vi "UEvent_MEASURE_SEQ1_CLEAN_UP_DAQ.vi"(6 "USB  in":tag, 9 "Vout  - Vbat profile":enum16{"3.8VDC", "2.9VDC", "By Pass", "4.0VDC"}(ring), 10 "Range - Shunts in":T1, 11 "TASK IN":refnum<k21>) -> (0 "error out":errorcluster, 1 "DevSerialNum":u32, 7 "Power ON/OFF":bool)   [LabVIEW 2015]
uses:
  Range_Shunt_selector.ctl
  <resource>/objmgr/daqmx.rc
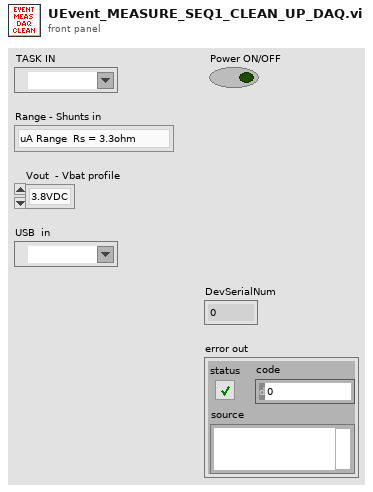
[diagram p1: front panel]
types:
  T1 = typedef "Range_Shunt_selector.ctl" = enum16{"uA Range  Rs = 3.3ohm", "mA Range Rs = 3.3ohm", "mA Range Rs = 1ohm", "mA Range Rs = 1ohm - X2"}
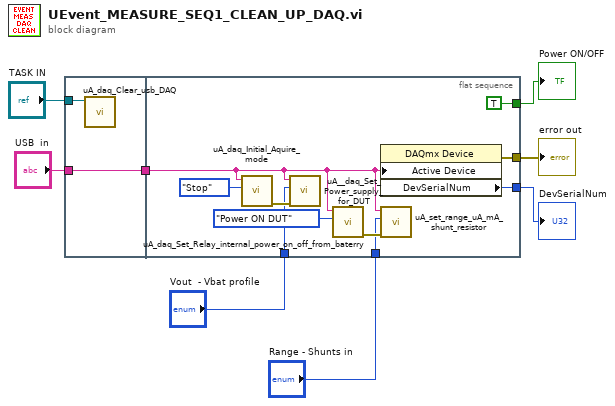
[diagram p0: block diagram]
diagram:
  n1 = flat-sequence {
    tunnel: "USB  in" -> [w10]
    tunnel: [w10] -> w8
    tunnel: "TASK IN" -> [w9]
    tunnel: w8 -> [w16]
    tunnel: [w17] -> w2
    tunnel: "Range - Shunts in" -> [w14]
    tunnel: "Vout  - Vbat profile" -> [w13]
    tunnel: [w12] -> w6
    tunnel: [TRUE ("Power ON/OFF")] -> w7
    frame #0 {
      n2 = call "uA_daq_Clear_usb_DAQ.vi"("Refnum in"=w9) -> ()  [unwired: 11 in]
    }
    frame #1 {
      n3 = call "uA_daq_Initial_Aquire_mode.vi"("Acquire Mode"=enum16{"Streaming", "Read All", "Stop"}."Stop", "USB DAQ"=w16) -> ("error out"=w18:errorcluster)  [unwired: 8 in, 1 out]
      n4 = call "uA__daq_Set_Power_supply_for_DUT.vi"("error in"=w18, "DUT Voltage Selector"=w13, "USB DAQ"=w16) -> ()  [unwired: 8 in, 1 out]
      n5 = call "uA_daq_Set_Relay_internal_power_on_off_from_baterry.vi"("Power ON/OFF DUT"=enum16{"Power ON DUT", "Power OFF DUT"}."Power ON DUT", "USB DAQ"=w16) -> ("error out"=w15:errorcluster)  [unwired: 9 in]
      n6 = property class="DAQmx Device"("Active Device"=w16) -> (error out=w17:errorcluster, "DevSerialNum"=w12:u32)  [unwired: 2 in, 1 out]
      n7 = call "uA_set_range_uA_mA_shunt_resistor.vi"("error in"=w15, "Range - Shunts"=w14, "device name"=w16) -> ()  [unwired: 8 in, 1 out]
    }
  }
  "Power ON/OFF" <- w7
  "DevSerialNum" <- w6
  "error out" <- w2
